vi "Button2ToggleV2.0.vi"(9 "a":bool, 10 "fNodeA(in)":bool, 11 "fNodeB":bool) -> (1 "Result(clone)":bool, 2 "fNodeA(out)":bool, 3 "Latched Bool (+fNodeB)":bool)   [LabVIEW 2013]
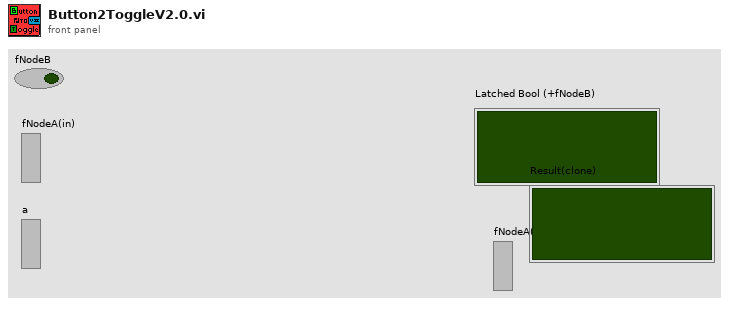
[diagram p1: front panel]
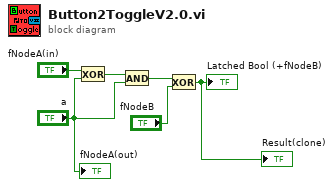
[diagram p0: block diagram]
diagram:
  n1 = Exclusive Or(1:"a", 2:"fNodeA(in)") -> (0:w5:bool)
  n2 = And(x=w5, y="a") -> (x .and. y?=w4:bool)
  n3 = Exclusive Or(1:"fNodeB", 2:w4) -> (0:→"Latched Bool (+fNodeB)" →"Result(clone)":bool)
  "fNodeA(out)" <- "a"
